vi "UpdatePanels.vi"(8 "error in (no error)":errorcluster, 11 "Bouncer in":refnum<class "Bouncer.lvclass">) -> (0 "error out":errorcluster, 3 "Game out":refnum<class "Bouncer.lvclass">)   [LabVIEW 2019, in "RT_Game.lvlib" / "Bouncer.lvclass"]
uses:
  Bouncer.lvclass
  C:/Users/FreshBob/Dropbox/VIs/myRIO_GameConsole/RT/RT_Game/Game/Game.lvclass
  Game/Game.lvclass/Game.ctl
  Bouncer.lvclass/Bouncer.ctl
  Game/Read Singleplayer.vi
  PongPanel/PongPanel.lvclass
  Game/Game.lvclass
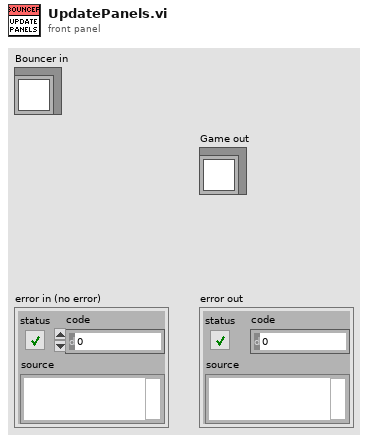
[diagram p1: front panel]
types:
  T1 = cluster{"Controls_1":cluster{"DirectionX":i8, "DirectionY":i8, "Button1":bool, "Button2":bool}, "Controls_2":cluster{"DirectionX":i8, "DirectionY":i8, "Button1":bool, "Button2":bool}, "SystemButton":bool}
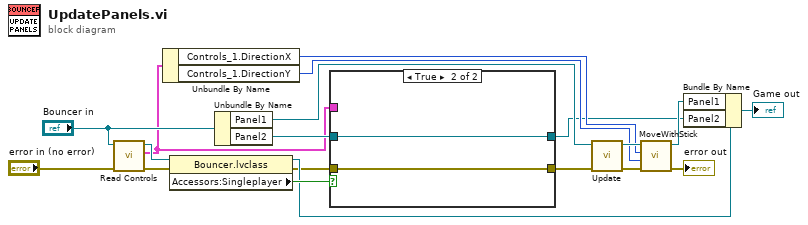
[diagram p0: block diagram]
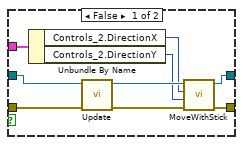
[diagram p2: hidden frame]
diagram:
  n1 = call "Read Controls.vi"("error in (no error)"="error in (no error)", "Game in"="Bouncer in") -> ("error out"=w5:errorcluster, "Controls"=w12:T1, "Game out"=w14:refnum<class "Bouncer.lvclass">)  [unwired: 7 in]
  n2 = Unbundle By Name(w12) -> ("Controls_1.DirectionX"=w6:i8, "Controls_1.DirectionY"=w7:i8)
  n3 = property class="Bouncer.lvclass"(reference=w14, error in=w5) -> (reference out=w15:refnum<class "Bouncer.lvclass">, error out=w13:errorcluster, "Accessors:Singleplayer"=w16:bool)
  n4 = Unbundle By Name("Bouncer in") -> ("Panel1"=w18:refnum<class "PongPanel.lvclass">, "Panel2"=w19:refnum<class "PongPanel.lvclass">)
  n5 = case shown="True" w16 {
    tunnel: w13 -> [w28 w30]
    tunnel: w19 -> [w26 w29]
    tunnel: [w25 w30] -> w11
    tunnel: w12 -> [w23 _]
    tunnel: [w20 w29] -> w1
    frame False {
      n6 = Unbundle By Name(w23) -> ("Controls_2.DirectionX"=w22:i8, "Controls_2.DirectionY"=w21:i8)
      n7 = call-dynamic "Update.vi"("error in (no error)"=w28, "GameObject in"=w26) -> ("error out"=w27:errorcluster, "GameObject out"=w24:refnum<class "PongPanel.lvclass">)  [unwired: 8 in]
      n8 = call "MoveWithStick.vi"("error in (no error)"=w27, "DirectionY"=w21, "DirectionX"=w22, "PongPanel in"=w24) -> ("error out"=w25:errorcluster, "PongPanel out"=w20:refnum<class "PongPanel.lvclass">)  [unwired: 6 in]
    }
    frame True {
    }
  }
  n9 = call-dynamic "Update.vi"("error in (no error)"=w11, "GameObject in"=w18) -> ("error out"=w9:errorcluster, "GameObject out"=w10:refnum<class "PongPanel.lvclass">)  [unwired: 8 in]
  n10 = call "MoveWithStick.vi"("error in (no error)"=w9, "DirectionY"=w7, "DirectionX"=w6, "PongPanel in"=w10) -> ("error out"=→"error out":errorcluster, "PongPanel out"=w2:refnum<class "PongPanel.lvclass">)  [unwired: 6 in]
  n11 = Bundle By Name(cluster=w15, "Panel1"=w2, "Panel2"=w1) -> (→"Game out":refnum<class "Bouncer.lvclass">)
